vi "Pascal Case to Standard.vi"(8 "error in (no error)":errorcluster, 11 "Input String":string) -> (0 "error out":errorcluster, 3 "Output String":string)   [LabVIEW 2015, in "Case Manipulation.lvlib"]
doc: "Introduction:\nWe often remove the spaces between words because programs of different sorts reserve the space (‘ ’) character for special purposes. Because the space character is reserved, we cannot use it to represent a concept that we express in our human language with multiple words.\nPascal Case:\nThis is also a very popular way to combine words to form a single concept. It is often used as a convention in declaring classes in many languages."
uses:
  Case Manipulation.lvlib
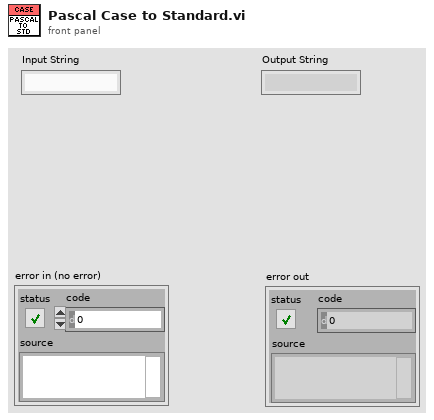
[diagram p1: front panel]
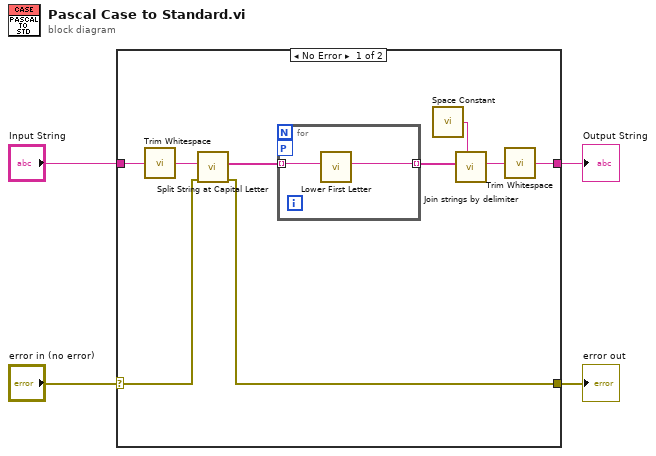
[diagram p0: block diagram]
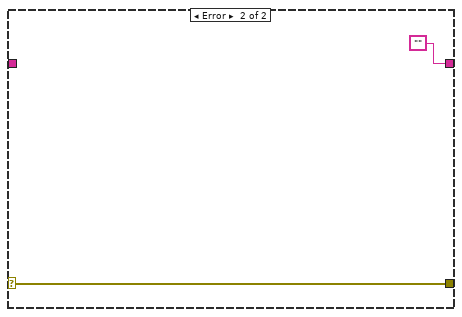
[diagram p2: hidden frame]
diagram:
  n1 = case shown="No Error" "error in (no error)" {
    selector: "error in (no error)" -> [w11 w16]
    tunnel: [w7 w16] -> w2
    tunnel: [w6 ""] -> w3
    tunnel: "Input String" -> [w13 _]
    frame No Error {
      n2 = call <vilib>:"Trim Whitespace.vi"("string"=w13) -> ("trimmed string"=w5:string)  [unwired: 1 in]
      n3 = call "Split String at Capital Letter.vi"("error in (no error)"=w11, "String In"=w5) -> ("error out"=w7:errorcluster, "String Array Out"=w12:string[])  [unwired: 8 in]
      n4 = for {
        tunnel: w12 -> [w15] mode=indexing
        tunnel: [w14] -> w10 mode=indexing
        workers-P: _ -> [_]
        n5 = call "Lower First Letter.vi"("String In"=w15) -> ("String Out"=w14:string)  [unwired: 10 in]
      }
      n6 = call <vilib>:"Space Constant.vi"() -> ("String"=w9:string)
      n7 = call "Join strings by delimiter.vi"("Delimiter"=w9, "Strings []"=w10) -> ("String Out"=w8:string)  [unwired: 9 in]
      n8 = call <vilib>:"Trim Whitespace.vi"("string"=w8) -> ("trimmed string"=w6:string)  [unwired: 1 in]
    }
    frame Error {
    }
  }
  "error out" <- w2
  "Output String" <- w3
